vi "Background Loop Step.vi"(8 "error in (no error)":errorcluster, 10 "Action":T1, 11 "DAQmx Lockin Digitizer Driver in":refnum<class "DAQmx Lockin Digitizer Driver.lvclass">) -> (0 "error out":errorcluster, 1 "Next step delay":i32, 2 "Action out":T1, 3 "DAQmx Lockin Digitizer Driver out":refnum<class "DAQmx Lockin Digitizer Driver.lvclass">, 4 "Result":refnum<class "Acquired Result.lvclass">)   [LabVIEW 2021, in "DAQmx Lockin Digitizer Driver.lvclass"]
uses:
  DAQmx Lockin Digitizer Driver.lvclass
  C:/GitHub/NHMFL_Core/Libraries/Instruments/Pulse Driver/Lockin Digitizer Driver/Lockin Digitizer Driver.lvclass
  C:/GitHub/NHMFL_Core/Libraries/Instruments/Pulse Driver/Pulse Driver.lvclass
  C:/GitHub/NHMFL_Core/Libraries/NI-DAQ/DAQmx Digitizer/DAQmx Digitizer.lvclass
  LabActor/Worker/Worker Actor/Background Loop Action.ctl
  Instruments/Results/Acquired Result/Acquired Result.lvclass
  LabActor/Controllers/Process Controller/Request type.ctl
  Instruments/Pulse Driver/Pulse Driver.lvclass/Pulse Driver.ctl
  DAQmx Lockin Digitizer Driver.lvclass/DAQmx Lockin Digitizer Driver.ctl
  Instruments/Pulse Driver/Lockin Digitizer Driver/Lockin Digitizer Driver.lvclass/Lockin Digitizer Driver.ctl
  <vilib>/DAQmx/write.llb/DAQmx Write (Analog 2D DBL NChan NSamp).vi
  <vilib>/DAQmx/read.llb/DAQmx Read (Analog 2D DBL NChan NSamp).vi
  Instruments/Pulse Driver/Read Samples per read.vi
  Instruments/Pulse Driver/Read Samples per channel.vi
  Instruments/Pulse Driver/Lockin Digitizer Driver/Write Input buffer.vi
  Instruments/Pulse Driver/Lockin Digitizer Driver/Write Output buffer.vi
  <vilib>/DAQmx/miscellaneous.llb/DAQmx Fill In Error Info.vi
  <vilib>/Analysis/NI_AALBase.lvlib
  <resource>/objmgr/daqmx.rc
panel:
  out "sleep time":u32
  out "millisecond timer value":u32
  out "elapsed time":u32
  out "Result ready":bool
  out "Armed":bool
  out "Recording compleste":bool
  out "AI Task":string
  out "AO task":string
  out "call chain":string[](array[string])
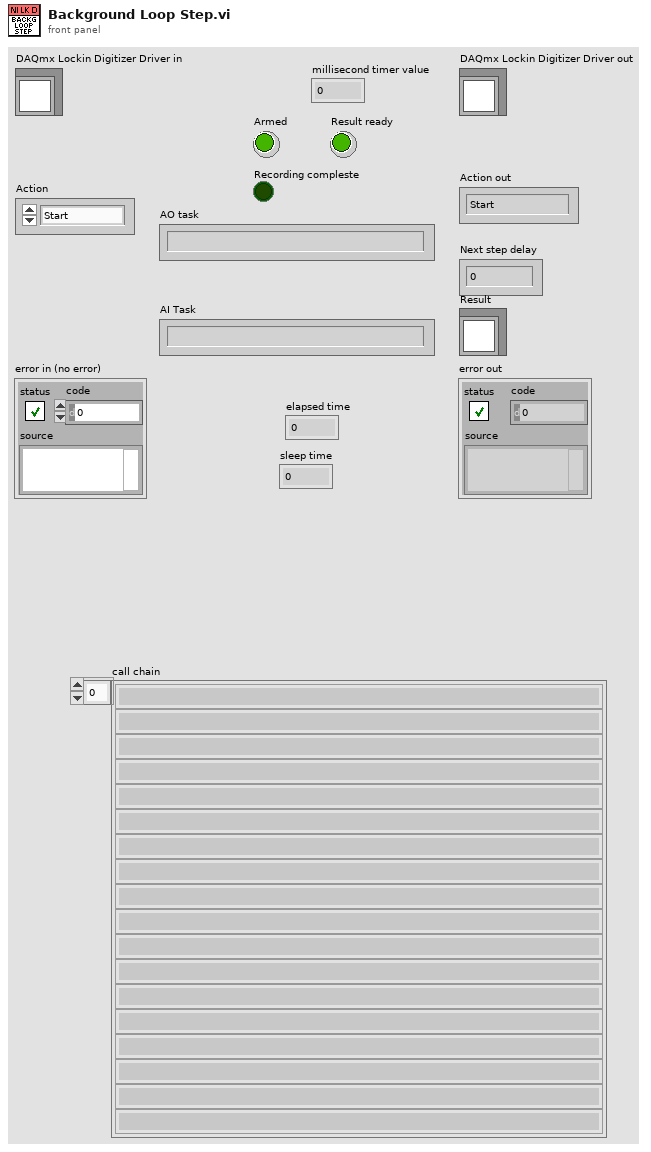
[diagram p1: front panel]
types:
  T1 = typedef "Background Loop Action.ctl" = enum16{"Start", "Continue", "Stop"}
  T2 = typedef "Request type.ctl" = enum16{"Process complete", "User command", "Auto-restart", "Error"}
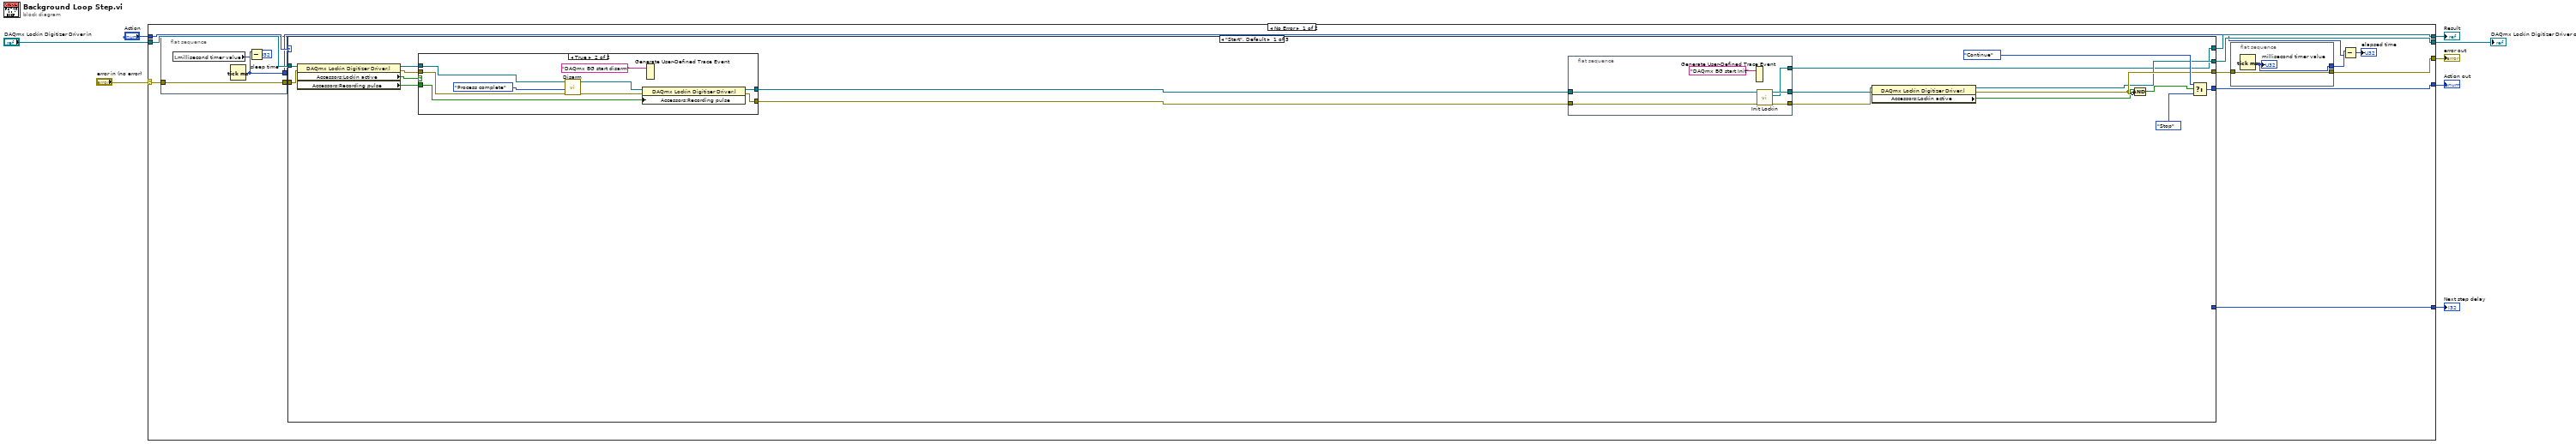
[diagram p0: block diagram]
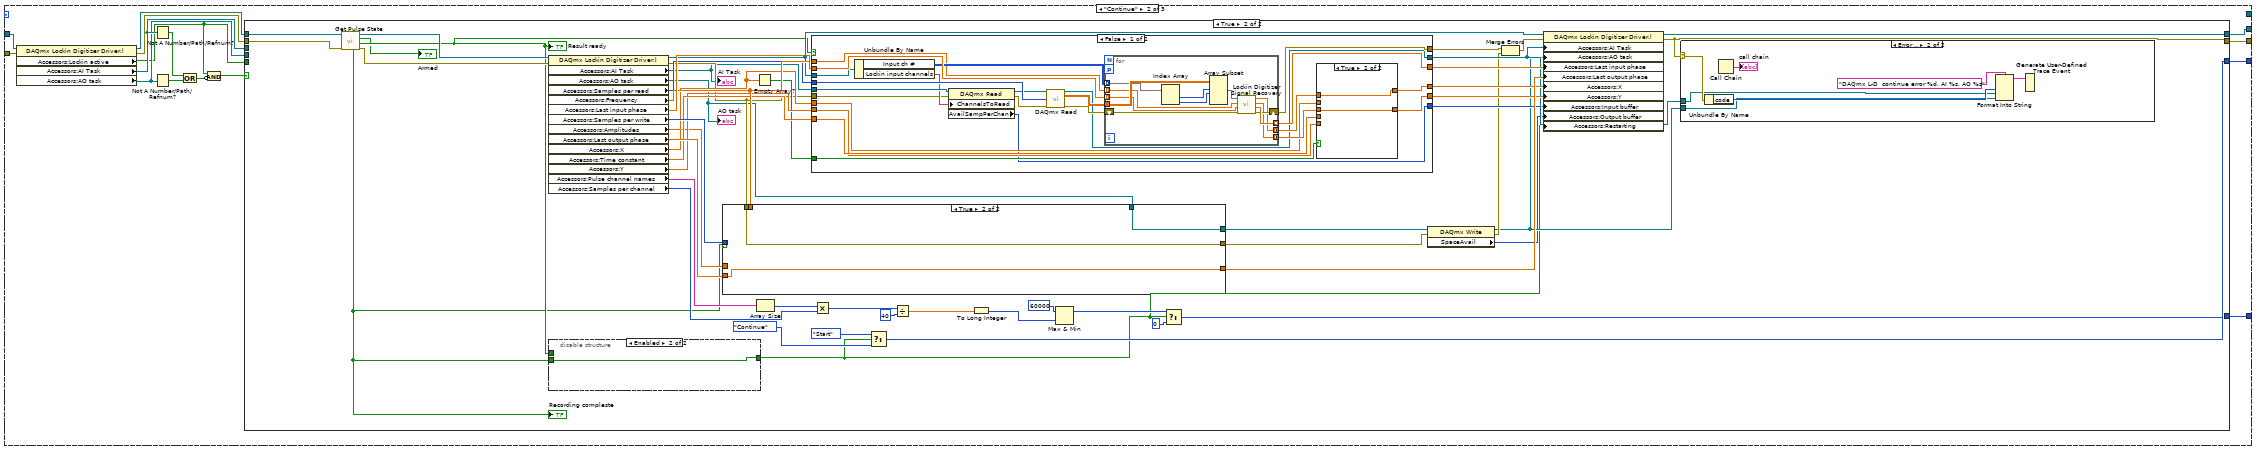
[diagram p3: hidden frame]
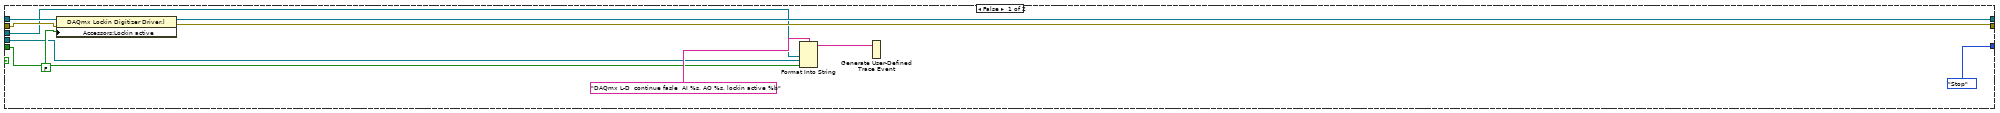
[diagram p4: hidden frame]
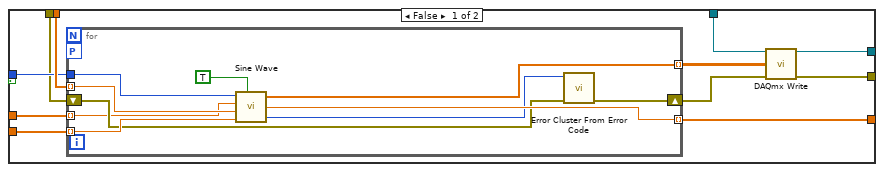
[diagram p5: hidden frame]
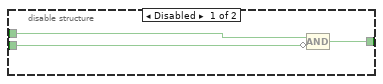
[diagram p6: hidden frame]
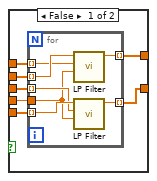
[diagram p7: hidden frame]
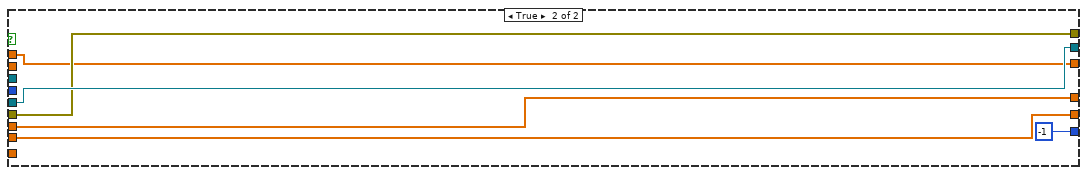
[diagram p8: hidden frame]
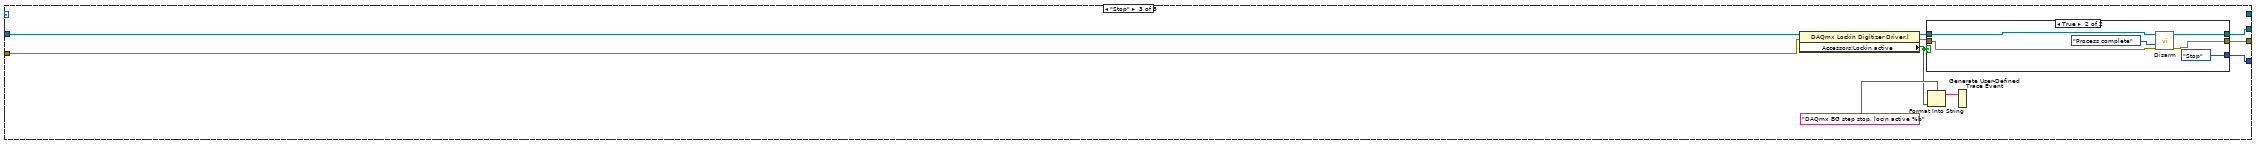
[diagram p10: hidden frame]
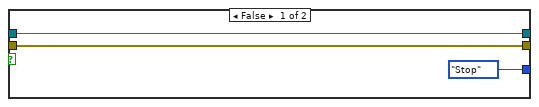
[diagram p11: hidden frame]
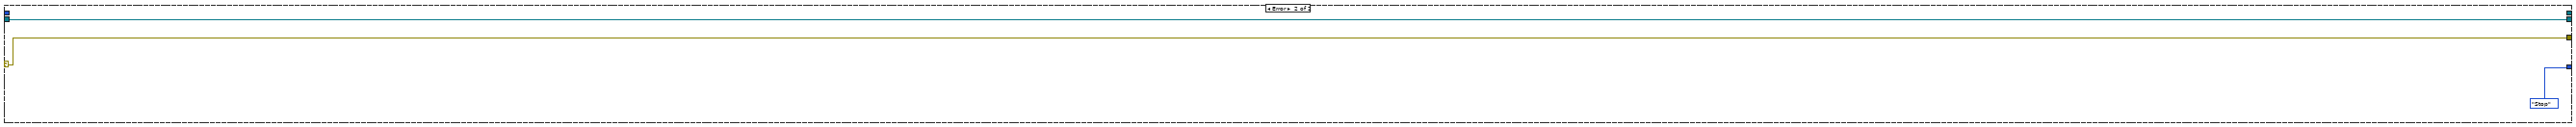
[diagram p12: hidden frame]
diagram:
  n1 = case shown="No Error" "error in (no error)" {
    selector: "error in (no error)" -> [w15 w254]
    tunnel: [w12 w254] -> w7
    tunnel: [w21 w253] -> w5
    tunnel: "DAQmx Lockin Digitizer Driver in" -> [w20 w253]
    tunnel: "Action" -> [w19 _]
    tunnel: [w18 Background_Loop_Action."Stop" ("Action")] -> w3
    tunnel: [w17 _] -> w2
    tunnel: [w16 _] -> w1
    frame No Error {
      n2 = flat-sequence {
        tunnel: w15 -> [w27]
        tunnel: [w27] -> w14
        tunnel: [w26] -> w10
        frame #0 {
          n3 = local read "millisecond timer value"() -> (w25:u32)
          n4 = Tick Count (ms)() -> (millisecond timer value=w26:u32)
          n5 = Subtract(x=w26, y=w25) -> (x-y=→"sleep time":u32)
        }
      }
      n6 = case shown="\"Start\", Default" w19 {
        tunnel: [w40 w77 w242] -> w13
        tunnel: [w38 w76 w241] -> w21
        tunnel: w14 -> [w32 w75 w237]
        tunnel: w20 -> [w30 w72 w239]
        tunnel: [w42 w74 w240] -> w18
        tunnel: [_ w63 _] -> w17
        tunnel: [w28 _ _] -> w16
        frame "Start", Default {
          n7 = property class="DAQmx Lockin Digitizer Driver.l"(reference=w30, error in=w32) -> (reference out=w36:refnum<class "DAQmx Lockin Digitizer Driver.lvclass">, error out=w34:errorcluster, "Accessors:Lockin active"=w35:bool, "Accessors:Recording pulse"=w29:bool)
          n8 = case shown="True" w35 {
            tunnel: w36 -> [w53 w60]
            tunnel: w34 -> [w52 w61]
            tunnel: [w52 w57] -> w33
            tunnel: [w53 w55] -> w31
            tunnel: w29 -> [_ w54]
            frame False {
            }
            frame True {
              n9 = call-dynamic "Disarm.vi"("error in (no error)"=w61, "Request type"=Request_type."Process complete", "DAQmx Lockin Digitizer Driver in"=w60) -> ("error out"=w59:errorcluster, "DAQmx Lockin Digitizer Driver out"=w56:refnum<class "DAQmx Lockin Digitizer Driver.lvclass">)  [unwired: 6 in, 1 out]
              n10 = Generate User-Defined Trace Event(2:"DAQmx BG start disarm" ("string")) -> ()  [unwired: 1 in]
              n11 = property class="DAQmx Lockin Digitizer Driver.l"(reference=w56, error in=w59, "Accessors:Recording pulse"=w54) -> (reference out=w55:refnum<class "DAQmx Lockin Digitizer Driver.lvclass">, error out=w57:errorcluster)
            }
          }
          n12 = flat-sequence {
            tunnel: [w51] -> w41
            tunnel: [w50] -> w39
            tunnel: w33 -> [w48]
            tunnel: w31 -> [w47]
            tunnel: [w46] -> w28
            frame #0 {
              n13 = Generate User-Defined Trace Event(2:"DAQmx BG start Init" ("string")) -> ()  [unwired: 1 in]
              n14 = call-dynamic "Init Lockin.vi"("error in (no error)"=w48, "DAQmx Lockin Digitizer Driver in"=w47) -> ("error out"=w51:errorcluster, "Result"=w46:refnum<class "Acquired Result.lvclass">, "DAQmx Lockin Digitizer Driver out"=w50:refnum<class "DAQmx Lockin Digitizer Driver.lvclass">)  [unwired: 7 in]
            }
          }
          n15 = property class="DAQmx Lockin Digitizer Driver.l"(reference=w39, error in=w41) -> (reference out=w38:refnum<class "DAQmx Lockin Digitizer Driver.lvclass">, error out=w40:errorcluster, "Accessors:Lockin active"=w37:bool)
          n16 = Compound Arithmetic op=AND(w37, invert w40) -> (w45:bool)
          n17 = Select(t=Background_Loop_Action."Continue" ("Action"), s=w45, f=Background_Loop_Action."Stop" ("Action")) -> (s? t:f=w42:T1)
        }
        frame "Continue" {
          n18 = property class="DAQmx Lockin Digitizer Driver.l"(reference=w72, error in=w75) -> (reference out=w71:refnum<class "DAQmx Lockin Digitizer Driver.lvclass">, error out=w73:errorcluster, "Accessors:Lockin active"=w64:bool, "Accessors:AI Task"=w66:refnum<k21>, "Accessors:AO task"=w65:refnum<k21>)
          n19 = Not A Number/Path/Refnum?(number/path/refnum=w66) -> (NaN/Path/Refnum?=w70:bool)
          n20 = Not A Number/Path/Refnum?(number/path/refnum=w65) -> (NaN/Path/Refnum?=w69:bool)
          n21 = Or(x=w70, y=w69) -> (x .or. y?=w67:bool)
          n22 = Compound Arithmetic op=AND(w64, invert w67) -> (w68:bool)
          n23 = case shown="True" w68 {
            tunnel: [w86 w120] -> w77
            tunnel: [w84 w131] -> w76
            tunnel: w73 -> [w85 w117]
            tunnel: w71 -> [w83 w118]
            tunnel: [Background_Loop_Action."Stop" ("Action") w111] -> w74
            tunnel: w66 -> [w80 _]
            tunnel: w65 -> [w79 _]
            tunnel: w64 -> [w78 _]
            tunnel: [_ w109] -> w63
            frame False {
              n24 = property class="DAQmx Lockin Digitizer Driver.l"(reference=w83, error in=w85, "Accessors:Lockin active"=FALSE ("Lockin active")) -> (reference out=w84:refnum<class "DAQmx Lockin Digitizer Driver.lvclass">, error out=w86:errorcluster)
              n25 = Format Into String(format string="DAQmx L-D  continue fasle  AI %s, AO %s, lockin active %b" ("string"), w80, w79, w78) -> (resulting string=w81:string)  [unwired: 2 in, 1 out]
              n26 = Generate User-Defined Trace Event(2:w81) -> ()  [unwired: 1 in]
            }
            frame True {
              n27 = call-dynamic "Get Pulse State.vi"("error in (no error)"=w117, "DAQmx Digitizer in"=w118) -> ("error out"=w116:errorcluster, "Result ready"=w113:bool, "Armed"=→"Armed":bool, "DAQmx Digitizer out"=w115:refnum<class "DAQmx Lockin Digitizer Driver.lvclass">, "Recording compleste"=w89:bool)  [unwired: 5 in]
              "Recording compleste" <- w89
              "Result ready" <- w113
              n28 = property class="DAQmx Lockin Digitizer Driver.l"(reference=w115, error in=w116) -> (reference out=w132:refnum<class "DAQmx Lockin Digitizer Driver.lvclass">, error out=w121:errorcluster, "Accessors:AI Task"=w92:refnum<k21>, "Accessors:AO task"=w93:refnum<k21>, "Accessors:Samples per read"=w126:i32, "Accessors:Frequency"=w138:dbl[], "Accessors:Last input phase"=w139:dbl[], "Accessors:Samples per write"=w137:i32, "Accessors:Amplitudes"=w122:dbl[], "Accessors:Last output phase"=w135:dbl[], "Accessors:X"=w124:dbl[], "Accessors:Time constant"=w128:dbl, "Accessors:Y"=w127:dbl[], "Accessors:Pulse channel names"=w101:string[], "Accessors:Samples per channel"=w99:i32)
              "AO task" <- w93
              "AI Task" <- w92
              n29 = disable-structure shown="Enabled" {
                disable-tunnel: w113 -> [w166 _]
                disable-tunnel: [w165 w167] -> w90
                disable-tunnel: w89 -> [w164 w167]
                frame Disabled {
                  n30 = Compound Arithmetic op=AND(w166, invert w164) -> (w165:bool)
                }
                frame Enabled {
                }
              }
              n31 = case shown="True" w89 {
                tunnel: w138 -> [w150 _]
                tunnel: w137 -> [w149 _]
                tunnel: [w148 w161] -> w136
                tunnel: w135 -> [w146 w161]
                tunnel: w122 -> [w144 _]
                tunnel: w121 -> [w143 w162]
                tunnel: [w142 w163] -> w106
                tunnel: [w141 w162] -> w105
                tunnel: w93 -> [w140 w163]
                frame False {
                  n32 = for {
                    tunnel: w150 -> [w160] mode=indexing
                    tunnel: w149 -> [w157]
                    tunnel: w146 -> [w159] mode=indexing
                    tunnel: [w158] -> w148 mode=indexing
                    tunnel: [w156] -> w147 mode=indexing
                    shift-right: [w152] -> w145
                    shift-left: w143 -> [w153]
                    workers-P: _ -> [_]
                    tunnel: w144 -> [w151] mode=indexing
                    n33 = call <vilib>:"Sine Wave.vi"("samples"=w157, "amplitude"=w151, "frequency"=w160, "phase in"=w159, "reset phase"=TRUE) -> ("sine wave"=w156:dbl[], "phase out"=w158:dbl, "error"=w154:i32)
                    n34 = call <vilib>:"Error Cluster From Error Code.vi"("error in (no error)"=w153, "error code (0)"=w154) -> ("error out"=w152:errorcluster)  [unwired: 7 in]
                  }
                  n35 = call-poly <vilib>:"DAQmx Write.vi"("task/channels in"=w140, "data"=w147, "error in"=w145) -> ("task out"=w142:refnum<k21>, "error out"=w141:errorcluster)  [unwired: 10 in, 1 out]
                }
                frame True {
                }
              }
              n36 = Empty Array?(array=w124) -> (empty?=w123:bool)
              n37 = Array Size(array=w101) -> (size(s)=w100:i32)
              n38 = case shown="False" w113 {
                tunnel: w139 -> [w190 _]
                tunnel: w138 -> [w188 w223]
                tunnel: [w187 w224] -> w134
                tunnel: w132 -> [w185 _]
                tunnel: [w182 w222] -> w130
                tunnel: [w181 w221] -> w129
                tunnel: w128 -> [w180 _]
                tunnel: w127 -> [w179 w221]
                tunnel: w126 -> [w178 _]
                tunnel: [w177 w223] -> w125
                tunnel: w92 -> [w176 w225]
                tunnel: w124 -> [w175 w222]
                tunnel: w123 -> [w174 _]
                tunnel: w121 -> [w172 w224]
                tunnel: [w169 w225] -> w119
                tunnel: [w168 i64 -1 ("AvailSampPerChan")] -> w107
                frame False {
                  n39 = Unbundle By Name(w185) -> ("Input ch #"=w189:i32[][], "Lockin input channels"=w173:string)
                  n40 = property class="DAQmx Read"(reference=w176, error in=w172, "ChannelsToRead"=w173) -> (reference out=w170:refnum<k21>, error out=w171:errorcluster, "AvailSampPerChan"=w168:u32)
                  n41 = call-poly <vilib>:"DAQmx Read.vi"("task/channels in"=w170, "number of samples per channel"=w178, "error in"=w171) -> ("task out"=w169:refnum<k21>, "data"=w191:dbl[][], "error out"=w186:errorcluster)  [unwired: 10 in]
                  n42 = for {
                    tunnel: w191 -> [w218]
                    tunnel: [w219] -> w177 mode=indexing
                    workers-P: _ -> [_]
                    tunnel: w188 -> [w216] mode=indexing
                    tunnel: w190 -> [w215] mode=indexing
                    tunnel: w189 -> [w214] mode=indexing
                    shift-right: [w211] -> w187
                    shift-left: w186 -> [w210]
                    tunnel: [w209] -> w184 mode=concatenating
                    tunnel: [w208] -> w183 mode=concatenating
                    n43 = Index Array(array=w214) -> (element #1=w213:i32, element #2=w212:i32)  [unwired: 2 in]
                    n44 = Array Subset(array=w218, index (row)=w213, length (row)=w212) -> (w217:dbl[][])  [unwired: 2 in]
                    n45 = call "Lockin Digitizer Signal Recovery.vi"("error in"=w210, "Phase in"=w215, "Frequency"=w216, "Input data"=w217) -> ("error out"=w211:errorcluster, "Phase out"=w219:dbl, "Y"=w208:dbl[], "X"=w209:dbl[])  [unwired: 4 in]
                  }
                  n46 = case shown="True" w174 {
                    tunnel: w184 -> [w198 w207]
                    tunnel: w183 -> [w197 w206]
                    tunnel: [w196 w207] -> w182
                    tunnel: [w195 w206] -> w181
                    tunnel: w180 -> [w194 _]
                    tunnel: w175 -> [w193 _]
                    tunnel: w179 -> [w192 _]
                    frame False {
                      n47 = for {
                        tunnel: w194 -> [w201]
                        tunnel: w193 -> [w205] mode=indexing
                        tunnel: w198 -> [w204] mode=indexing
                        tunnel: w192 -> [w203] mode=indexing
                        tunnel: w197 -> [w202] mode=indexing
                        tunnel: [w200] -> w196 mode=indexing
                        tunnel: [w199] -> w195 mode=indexing
                        n48 = call "LP Filter.vi"("Time constant"=w201, "New data"=w204, "Previous data"=w205) -> ("Filtered data"=w200:dbl)  [unwired: 8 in]
                        n49 = call "LP Filter.vi"("Time constant"=w201, "New data"=w202, "Previous data"=w203) -> ("Filtered data"=w199:dbl)  [unwired: 8 in]
                      }
                    }
                    frame True {
                    }
                  }
                }
                frame True {
                }
              }
              n50 = Multiply(x=w100, y=w99) -> (x*y=w98:i32)
              n51 = Select(t=Background_Loop_Action."Start" ("Action"), s=w90, f=Background_Loop_Action."Continue" ("Action")) -> (s? t:f=w111:T1)
              n52 = Divide(x=w98, y=40) -> (x/y=w95:dbl)
              n53 = To Long Integer(number=w95) -> (32bit integer=w94:i32)
              n54 = Max & Min(x=60000 ("Next step delay"), y=w94) -> (max(x,y)=w96:i32)  [unwired: 1 out]
              n55 = Select(t=w96, s=w90, f=0 ("Next step delay")) -> (s? t:f=w109:i32)
              n56 = property class="DAQmx Write"(reference=w106, error in=w105) -> (reference out=w103:refnum<k21>, error out=w104:errorcluster, "SpaceAvail"=w102:u32)
              n57 = Merge Errors(w134, w104) -> (w133:errorcluster)
              n58 = property class="DAQmx Lockin Digitizer Driver.l"(reference=w132, error in=w133, "Accessors:AI Task"=w119, "Accessors:AO task"=w103, "Accessors:Last input phase"=w125, "Accessors:Last output phase"=w136, "Accessors:X"=w130, "Accessors:Y"=w129, "Accessors:Input buffer"=w107, "Accessors:Output buffer"=w102, "Accessors:Restarting"=w90) -> (reference out=w131:refnum<class "DAQmx Lockin Digitizer Driver.lvclass">, error out=w120:errorcluster)
              n59 = case shown="Error .." w120 {
                selector: w120 -> [_ w232]
                tunnel: w119 -> [_ w228]
                tunnel: w103 -> [_ w227]
                frame No Error {
                }
                frame Error {
                  n60 = Unbundle By Name(w232) -> ("code"=w229:i32)
                  n61 = Call Chain() -> (call chain=→"call chain":string[])
                  n62 = Format Into String(format string="DAQmx L-D  continue error %d, AI %s, AO %s" ("string"), w229, w228, w227) -> (resulting string=w230:string)  [unwired: 2 in, 1 out]
                  n63 = Generate User-Defined Trace Event(2:w230) -> ()  [unwired: 1 in]
                }
              }
            }
          }
        }
        frame "Stop" {
          n64 = property class="DAQmx Lockin Digitizer Driver.l"(reference=w239, error in=w237) -> (reference out=w236:refnum<class "DAQmx Lockin Digitizer Driver.lvclass">, error out=w238:errorcluster, "Accessors:Lockin active"=w233:bool)
          n65 = case shown="True" w233 {
            tunnel: [w244 w249] -> w242
            tunnel: [w245 w247] -> w241
            tunnel: w238 -> [w244 w250]
            tunnel: w236 -> [w245 w248]
            tunnel: [Background_Loop_Action."Stop" ("Action") Background_Loop_Action."Stop" ("Action")] -> w240
            frame False {
            }
            frame True {
              n66 = call-dynamic "Disarm.vi"("error in (no error)"=w250, "Request type"=Request_type."Process complete", "DAQmx Lockin Digitizer Driver in"=w248) -> ("error out"=w249:errorcluster, "DAQmx Lockin Digitizer Driver out"=w247:refnum<class "DAQmx Lockin Digitizer Driver.lvclass">)  [unwired: 6 in, 1 out]
            }
          }
          n67 = Format Into String(format string="DAQmx BG step stop, locin active %b" ("string"), w233) -> (resulting string=w235:string)  [unwired: 2 in, 1 out]
          n68 = Generate User-Defined Trace Event(2:w235) -> ()  [unwired: 1 in]
        }
      }
      n69 = flat-sequence {
        tunnel: w13 -> [w23]
        tunnel: [w23] -> w12
        tunnel: [w22] -> w11
        frame #0 {
          n70 = Tick Count (ms)() -> (millisecond timer value=w22:u32)
          "millisecond timer value" <- w22
        }
      }
      n71 = Subtract(x=w11, y=w10) -> (x-y=→"elapsed time":u32)
    }
    frame Error {
    }
  }
  "error out" <- w7
  "DAQmx Lockin Digitizer Driver out" <- w5
  "Action out" <- w3
  "Next step delay" <- w2
  "Result" <- w1
